vi "SA_TRG_GET-MKR.vi"(8 "error in":errorcluster {"code" format="%.0x"}, 11 "Session In":refnum<visa-resource-name>="GPIB0::16::INSTR") -> (0 "error out":errorcluster {"code" format="%.0x"}, 2 "Ampl":dbl, 3 "Session Out":refnum<visa-resource-name>)   [LabVIEW 2018]
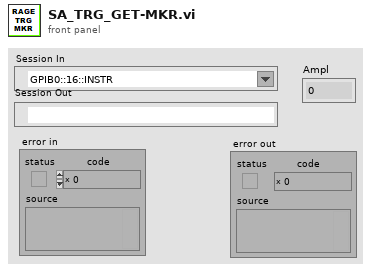
[diagram p1: front panel]
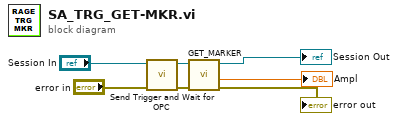
[diagram p0: block diagram]
diagram:
  n1 = call "Send Trigger and Wait for OPC.vi"("error in"="error in", "Session In"="Session In") -> ("error out"=w7:errorcluster, "Session Out"=w6:refnum<visa-resource-name>)  [unwired: 7 in, 1 out]
  n2 = call "GET_MARKER.vi"("error in"=w7, "Session In"=w6) -> ("error out"=→"error out":errorcluster, "Ampl_corr"=→"Ampl":dbl, "Session Out"=→"Session Out":refnum<visa-resource-name>)  [unwired: 6 in, 1 out]
